vi "Update_Error.vi"(8 "error in (no error)":errorcluster, 9 "Error?":i8, 10 "PV-URL":string, 11 "CS++Motor in":refnum<class "CS++Motor.lvclass">) -> (0 "error out":errorcluster, 3 "CS++Motor out":refnum<class "CS++Motor.lvclass">)   [LabVIEW 2015, in "CS++Motor.lvlib" / "CS++Motor.lvclass"]
doc: "This VI is executed via the corresponding Monitor Actor and delivers the information wether an axis shows an error or not."
uses:
  CS++Motor.lvclass
  <vilib>/event_ctls.llb/usereventprio.ctl
  CS++Motor.lvclass/CS++Motor.ctl
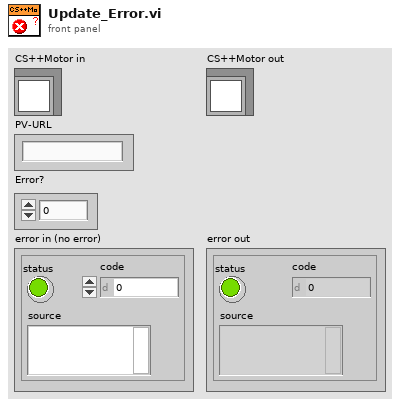
[diagram p1: front panel]
types:
  T1 = typedef "usereventprio.ctl" = enum32{"high priority", "normal priority"}
  T2 = cluster{"Command":string, "AxisNumber":u8, "Data":variant}
  T3 = cluster{"Update-Msg Name":string, "Update-Msg URLs":string[]}[]
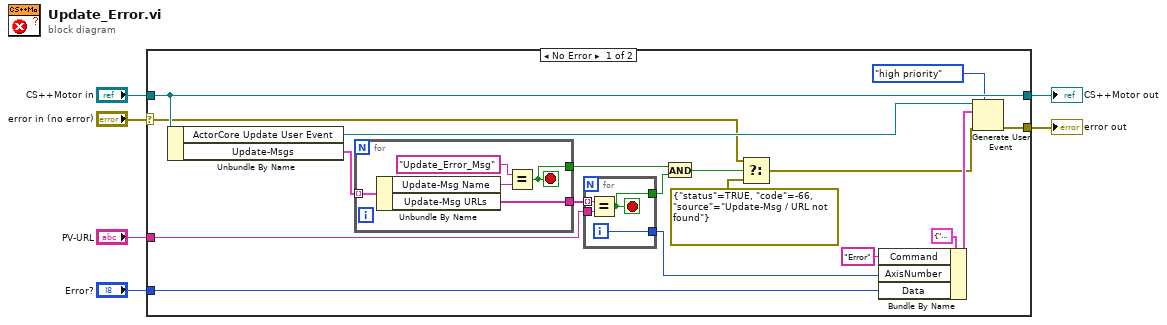
[diagram p0: block diagram]
diagram:
  n1 = case shown="No Error" "error in (no error)" {
    selector: "error in (no error)" -> [w10 w35]
    tunnel: [w22 w35] -> w5
    tunnel: [w17 w34] -> w3
    tunnel: "CS++Motor in" -> [w17 w34]
    tunnel: "Error?" -> [w20 _]
    tunnel: "PV-URL" -> [w15 _]
    frame No Error {
      n2 = Unbundle By Name(w17) -> ("ActorCore Update User Event"=w19:refnum<user-event>, "Update-Msgs"=w18:T3)
      n3 = for {
        tunnel: w18 -> [w33] mode=indexing
        tunnel: [w30] -> w16
        tunnel: [w29] -> w13
        stop <- w29 stop-if-true
        n4 = Unbundle By Name(w33) -> ("Update-Msg Name"=w32:string, "Update-Msg URLs"=w30:string[])
        n5 = Equal?(x="Update_Error_Msg", y=w32) -> (x = y?=w29:bool)
      }
      n6 = for {
        tunnel: w16 -> [w28] mode=indexing
        tunnel: w15 -> [w27]
        tunnel: [w26] -> w12
        tunnel: [w25] -> w14
        i -> [w25]
        stop <- w26 stop-if-true
        n7 = Equal?(x=w28, y=w27) -> (x = y?=w26:bool)
      }
      n8 = And(x=w13, y=w12) -> (x .and. y?=w11:bool)
      n9 = Select(t=w10, s=w11, f=errorcluster {"status"=TRUE, "code"=-66, "source"="Update-Msg / URL not found"}) -> (s? t:f=w9:errorcluster)
      n10 = Bundle By Name(cluster=T2 {"Command"="", "AxisNumber"=0, "Data"=variant} ("event data"), "Command"="Error", "AxisNumber"=w14, "Data"=w20) -> (w23:T2)
      n11 = Generate User Event(priority (normal)=usereventprio."high priority", user event=w19, event data cluster=w23, error in=w9) -> (error out=w22:errorcluster)  [unwired: 1 out]
    }
    frame Error {
    }
  }
  "error out" <- w5
  "CS++Motor out" <- w3
